vi "Rz.vi"(11 "theta":dbl) -> (3 "RotacionalZ":T1)   [LabVIEW 2011]
uses:
  <vilib>/Analysis/Matrix/Datatypes/RealMatrix.ctl
  <vilib>/Analysis/Matrix/NI_Matrix.lvlib
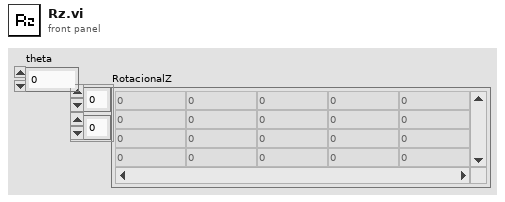
[diagram p1: front panel]
types:
  T1 = typedef "NI_Matrix.lvlib/RealMatrix.ctl" = dbl[][]
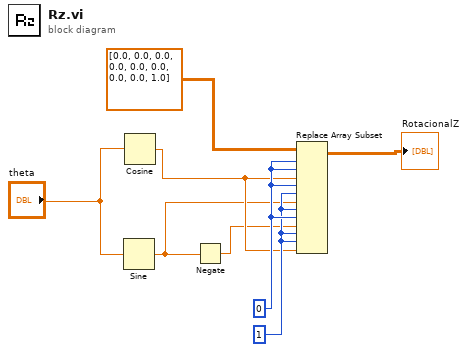
[diagram p0: block diagram]
diagram:
  w7 = 1
  w8 = 0
  n1 = Sine(x="theta") -> (sin(x)=w5:dbl)
  n2 = Cosine(x="theta") -> (cos(x)=w6:dbl)
  n3 = Negate(x=w5) -> (-x=w4:dbl)
  n4 = Replace Array Subset(array=T1 [[0.0, 0.0, 0.0], [0.0, 0.0, 0.0], [0.0, 0.0, 1.0]] ("Real Matrix"), new element #1=w6, index (row) #1=w8, index (col) #1=w8, new element #2=w5, index (row) #2=w8, index (col) #2=w7, new element #3=w4, index (row) #3=w7, index (col) #3=w8, new element #4=w6, index (row) #4=w7, index (col) #4=w7) -> (→"RotacionalZ":T1)
